vi "GetParam.vi"(8 "error in (no error)":errorcluster caption="entrée d'erreur (pas d'erreur)", 11 "Mutual_Info_Score.lvclass":refnum<class "Mutual_Info_Score.lvclass">) -> (0 "error out":errorcluster caption="sortie d'erreur", 2 "mutual_info_score":T1, 3 "Mutual_Info_Score.lvclass":refnum<class "Mutual_Info_Score.lvclass">)   [LabVIEW 2020, in "Mutual_Info_Score.lvclass"]
doc: "Get Parameters"
uses:
  Mutual_Info_Score.lvclass
  Mutual_Info_Score.lvclass/Mutual_Info_Score.ctl
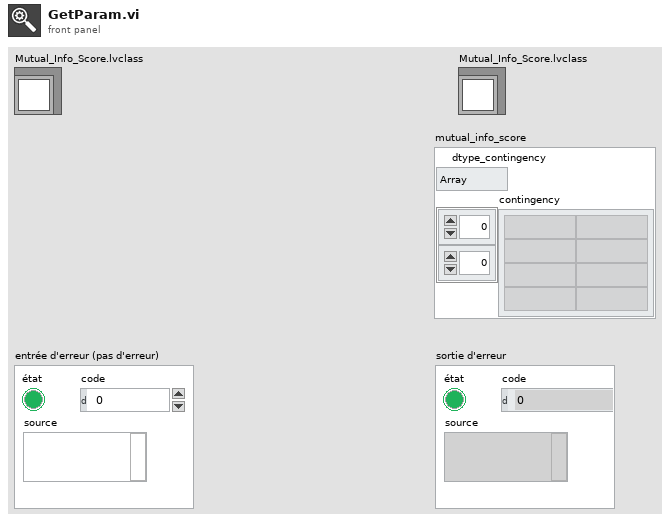
[diagram p1: front panel]
types:
  T1 = cluster{"dtype_contingency":enum16{"Array", "Sparse"}, "contingency":string[][]}
  T2 = cluster{"dtype_contingency":enum16{"Numeric Array", "String Array", "Sparse"}, "contingency":string[][]}
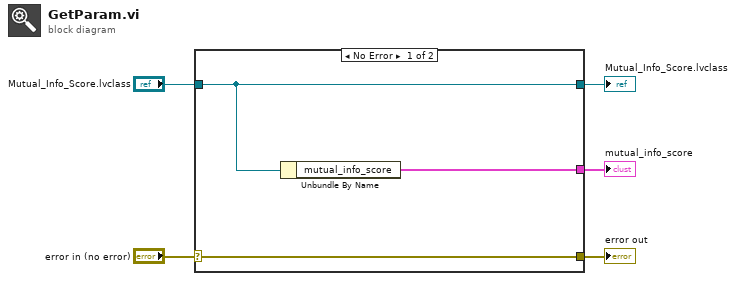
[diagram p0: block diagram]
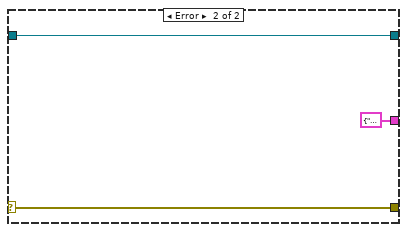
[diagram p2: hidden frame]
diagram:
  n1 = case shown="No Error" "error in (no error)" {
    selector: "error in (no error)" -> [w8 w10]
    tunnel: [w8 w10] -> w4
    tunnel: [w7 w11] -> w2
    tunnel: "Mutual_Info_Score.lvclass" -> [w7 w11]
    tunnel: [w6 T1 {"dtype_contingency"=enum."Array", "contingency"=[]} ("mutual_info_score")] -> w1
    frame No Error {
      n2 = Unbundle By Name(w7) -> ("mutual_info_score"=w6:T2)
    }
    frame Error {
    }
  }
  "error out" <- w4
  "Mutual_Info_Score.lvclass" <- w2
  "mutual_info_score" <- w1
